vi "ni579x Host Align.vi"(0 "sync.resources":T1, 1 "sync.meas.Reference Clock":refnum<k21>, 2 "sync.meas.FPGA I/O":refnum<k21>) -> (4 "sync.resources":T1)   [LabVIEW 2015, in "ni579x Synchronization v2 FPGA.lvlib"]
doc: "Align the targets participating in synchronization. This must occur before a signal can be synchronized.\n\nThere are two flavors of alignment to chose from -- Host Align and FPGA Align. The two flavors produce the same quality of synchronization, but differ in requirements and versatility of operation.\n\nWhen using <B>ni579x FPGA Align</B>, the Single Cycle Timed Loop (SCTL) rate (that this VI is in) must be an integer multiple of the <B>sync.cptr.Reference Clock</B> rate, and the SCTL clock must have a fixed phase relationship to the reference clock. Each target performs its alignment independently, so FPGA Align does not require a FPGA I/O line. It's also possible to use FPGA Align without host interaction. FPGA Align has 100% repeatability if-and-only-if the target-to-target phase relationship is low and does not change.\n\nWhen using <B>ni579x Host Align</B>, the SCTL rate may be arbitrary (yet still must have a fixed phase relationship to the other targets). The CPTR period may also be arbitrary. This alignment process is coordinated by the host, and requires an FPGA I/O line for orchestration. Host Align has 100% repeatability; if the hardware configuration remains constant, so will the level of synchronization.\n\n<B>Input Parameters</B>\n\n<B>sync.resources</B> identifies the Synchronization instance. 'sync.resources' is obtained from the ni579x Create VI of this library.\n\n<B>sync.meas.Reference Clock</B> is used by the measurement logic as the \"start\" signal. This is commonly PXI_Clk10.\n\n<B>sync.meas.FPGA I/O</B> is the FPGA I/O line that will be used to orchestrate starting the measurements. This is commonly a PXI Trig line.\n\nNote: For large NI chassis, make sure the PXI Trig line is routed to all bus segments that have targets participating in synchronization.\n\n<B>Output Parameters</B>\n\n<B>sync.resources</B> is the same instance that was passed in for 'sync.resources'."
uses:
  <instrlib>/ni579x/Synchronization/v2/FPGA/ni579x Synchronization v2 FPGA.lvlib
  <vilib>/eio/EIONode/EIONode.xnode
  <instrlib>/_niInstr/Basic Elements/v1/FPGA/niInstr Basic Elements v1 FPGA.lvlib
  <instrlib>/_niInstr/TDC/v1/FPGA/niInstr Overclocked TDC v1 FPGA.lvlib
  <vilib>/rvi/eio/common/nirviEmuTemplateMethod_errors.vi
  <instrlib>/ni579x/Synchronization/v2/FPGA/Implementation/Resources.ctl
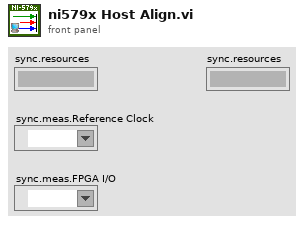
[diagram p1: front panel]
types:
  T1 = typedef "ni579x Synchronization v2 FPGA.lvlib/Resources.ctl" = cluster{"master":refnum<k21>, "meas.enable":refnum<k21>, "meas.ready":refnum<k21>, "meas.arm":refnum<k21>, "meas.valid":refnum<k21>, "meas.value":refnum<k21>, "meas.oversample clock":refnum<k21>, "meas.oversample factor":refnum<k21>, "cptr":refnum<k21>, "cptr.adjust":refnum<k21>, "cptr.period":refnum<k21>}
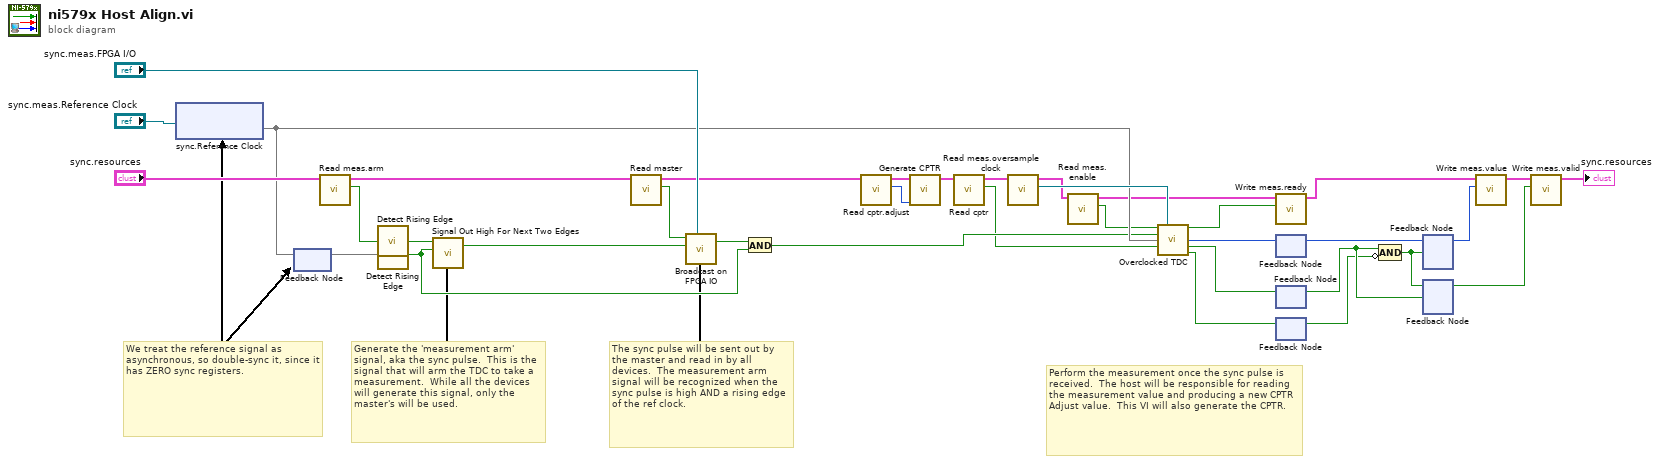
[diagram p0: block diagram]
diagram:
  # "We treat the reference signal as asynchronous, so double-sync it, since it has ZERO sync registers."
  # "Perform the measurement once the sync pulse is received.  The host will be responsible for reading the measurement value and producing a new CPTR Adjust value.  This VI will also generate the CPTR."
  # "The sync pulse will be sent out by the master and read in by all devices.  The measurement arm signal will be recognized when the sync pulse is high AND a rising edge of the ref clock."
  # "Generate the 'measurement arm' signal, aka the sync pulse.  This is the signal that will arm the TDC to take a measurement.  While all the devices will generate this signal, only the master's will be used."
  n1 = xnode ("sync.Reference Clock")("FPGA I/O In"="sync.meas.Reference Clock") -> ("I/O Item"=w14)  [unwired: 1 out]
  n2 = feedback #1() -> (w33)  [unwired: 1 in]
  n3 = feedback-in #1(w14) -> ()
  n4 = call <instrlib>:"Read meas.arm.vi"("sync.resources"="sync.resources") -> ("meas.arm"=w29:bool, "sync.resources"=w24:T1)  [unwired: 9 in]
  n5 = call <instrlib>:"Detect Rising Edge.vi"("signal"=w29) -> ("edge detected"=w34:bool)  [unwired: 14 in]
  n6 = call <instrlib>:"Detect Rising Edge.vi"("signal"=w33) -> ("edge detected"=w36:bool)  [unwired: 14 in]
  n7 = call <instrlib>:"Signal Out High For Next Two Edges.vi"("edge"=w36, "signal"=w34) -> ("signal for distribution"=w32:bool)  [unwired: 3 in]
  n8 = call <instrlib>:"Read master.vi"("sync.resources"=w24) -> ("master"=w28:bool, "sync.resources"=w21:T1)  [unwired: 9 in]
  n9 = call <instrlib>:"Broadcast on FPGA IO.vi"("FPGA I/O"="sync.meas.FPGA I/O", "signal in"=w32, "master"=w28) -> ("signal out"=w31:bool)  [unwired: 4 in]
  n10 = And(x=w31, y=w36) -> (x .and. y?=w8:bool)
  n11 = call <instrlib>:"Read cptr.adjust.vi"("sync.resources"=w21) -> ("cptr.adjust"=w20:u16, "sync.resources"=w22:T1)  [unwired: 9 in]
  n12 = call <instrlib>:"Generate CPTR.vi"("sync.cptr.adjust"=w20, "sync.resources"=w22) -> ("sync.resources"=w19:T1)  [unwired: 9 in]
  n13 = call <instrlib>:"Read cptr.vi"("sync.resources"=w19) -> ("cptr"=w7:bool, "sync.resources"=w16:T1)  [unwired: 9 in]
  n14 = call <instrlib>:"Read meas.oversample clock.vi"("sync.resources"=w16) -> ("meas.oversample clock"=w15:refnum<k21>, "sync.resources"=w13:T1)  [unwired: 9 in]
  n15 = call <instrlib>:"Read meas.enable.vi"("sync.resources"=w13) -> ("meas.enable"=w9:bool, "sync.resources"=w12:T1)  [unwired: 9 in]
  n16 = call <instrlib>:"Overclocked TDC.vi"("enable"=w9, "counter clock"=w15, "arm"=w8, "start"=w14, "stop"=w7) -> ("ready"=w11:bool, "count"=w6:u16, "count valid"=w5:bool, "rollover"=w4:bool)  [unwired: 6 in, 1 out]
  n17 = call <instrlib>:"Write meas.ready.vi"("meas.ready"=w11, "sync.resources"=w12) -> ("sync.resources"=w10:T1)  [unwired: 9 in]
  n18 = feedback #2() -> (w3:u16)  [unwired: 1 in]
  n19 = feedback-in #2(w6) -> ()
  n20 = feedback #3() -> (w2:bool)  [unwired: 1 in]
  n21 = feedback-in #3(w5) -> ()
  n22 = feedback #4() -> (w1:bool)  [unwired: 1 in]
  n23 = feedback-in #4(w4) -> ()
  n24 = Compound Arithmetic op=AND(w2, invert w1) -> (w27:bool)
  n25 = feedback #5() -> (w26:u16)  [unwired: 1 in]
  n26 = feedback-in #5(w3, w27) -> ()
  n27 = feedback #6() -> (w25:bool)  [unwired: 1 in]
  n28 = feedback-in #6(w27, w2) -> ()
  n29 = call <instrlib>:"Write meas.value.vi"("meas.value"=w26, "sync.resources"=w10) -> ("sync.resources"=w23:T1)  [unwired: 9 in]
  n30 = call <instrlib>:"Write meas.valid.vi"("meas.valid"=w25, "sync.resources"=w23) -> ("sync.resources"=→"sync.resources":T1)  [unwired: 9 in]
